vi "rsidr_core_global.vi"() -> ()   [LabVIEW 2020, in "Rohde&Schwarz RTx Oscilloscopes.lvlib"] (continued)
"Flags"=0, "Help"="Sets the transmission type to be triggered on.\n\nAvailable Repeated Capabilities:\nNone\n\nRemote-control command(s):\nTRIGger:A:MILStd:TTYPe"}, {"Level"=3, "Class Only"=FALSE, "Identifier"="RSRTX_ATTR_MILSTD_TRIGGER_FRAME", "Descriptive Name"="MILSTD Trigger Frame", "Data Type"=0, "Command"="TRIG:A:MILS:FRAM", "Access"=2, "Range Table"="RsRtx_rngMILSTDTriggerFrame", "Read Callback"="", "Write Callback"="", "Supported Models"="RTM|RTA", "Instrument Options"="", "Flags"=0, "Help"="Configures trigger frame.\n\nAvailable Repeated Capabilities:\nNone\n\nRemote-control command(s):\nTRIGger:A:MILStd:FRAMe"}, {"Level"=3, "Class Only"=TRUE, "Identifier"="", "Descriptive Name"="Error", "Data Type"=0, "Command"="", "Access"=0, "Range Table"="", "Read Callback"="", "Write Callback"="", "Supported Models"="", "Instrument Options"="", "Flags"=0, "Help"="Triggers on any combination of protocol errors. You can enable triggering on a specific type of error."}, {"Level"=4, "Class Only"=FALSE, "Identifier"="RSRTX_ATTR_MILSTD_TRIGGER_SYNCHRONIZATION_ERROR", "Descriptive Name"="MILSTD Trigger Synchronization Error", "Data Type"=3, "Command"="TRIG:A:MILS:ERR:SYNC", "Access"=2, "Range Table"="", "Read Callback"="", "Write Callback"="", "Supported Models"="RTM|RTA", "Instrument Options"="", "Flags"=0, "Help"="Enables/disables triggering when a sync impulse doesn&apos;t fulfil the technical requirements or when the transmission is not valid.\n\nAvailable Repeated Capabilities:\nNone\n\nRemote-control command(s):\nTRIGger:A:MILStd:ERRor:SYNC"}, {"Level"=4, "Class Only"=FALSE, "Identifier"="RSRTX_ATTR_MILSTD_TRIGGER_TIMEOUT_ERROR", "Descriptive Name"="MILSTD Trigger Timeout Error", "Data Type"=3, "Command"="TRIG:A:MILS:ERR:TIM", "Access"=2, "Range Table"="", "Read Callback"="", "Write Callback"="", "Supported Models"="RTM|RTA", "Instrument Options"="", "Flags"=0, "Help"="Enables/ disables triggering when the timeout is out of the set range.\n\nAvailable Repeated Capabilities:\nNone\n\nRemote-control command(s):\nTRIGger:A:MILStd:ERRor:TIMeout"}, {"Level"=4, "Class Only"=FALSE, "Identifier"="RSRTX_ATTR_MILSTD_TRIGGER_PARITY_ERROR", "Descriptive Name"="MILSTD Trigger Parity Error", "Data Type"=3, "Command"="TRIG:A:MILS:ERR:PAR", "Access"=2, "Range Table"="", "Read Callback"="", "Write Callback"="", "Supported Models"="RTM|RTA", "Instrument Options"="", "Flags"=0, "Help"="Enables/disables triggering when the parity is even.\n\nAvailable Repeated Capabilities:\nNone\n\nRemote-control command(s):\nTRIGger:A:MILStd:ERRor:PARity"}, {"Level"=4, "Class Only"=FALSE, "Identifier"="RSRTX_ATTR_MILSTD_TRIGGER_MANCHESTER_ERROR", "Descriptive Name"="MILSTD Trigger Manchester Error", "Data Type"=3, "Command"="TRIG:A:MILS:ERR:MANC", "Access"=2, "Range Table"="", "Read Callback"="", "Write Callback"="", "Supported Models"="RTM|RTA", "Instrument Options"="", "Flags"=0, "Help"="Enables/disables triggering if there is an error in the Manchester coding of the signal.\n\nAvailable Repeated Capabilities:\nNone\n\nRemote-control command(s):\nTRIGger:A:MILStd:ERRor:MANChester"}, {"Level"=3, "Class Only"=TRUE, "Identifier"="", "Descriptive Name"="Command", "Data Type"=0, "Command"="", "Access"=0, "Range Table"="", "Read Callback"="", "Write Callback"="", "Supported Models"="", "Instrument Options"="", "Flags"=0, "Help"="Triggers on any combination of protocol errors. You can enable triggering on a specific type of error."}, {"Level"=4, "Class Only"=FALSE, "Identifier"="RSRTX_ATTR_MILSTD_TRIGGER_COMMAND_TYPE", "Descriptive Name"="MILSTD Trigger Command Type", "Data Type"=0, "Command"="TRIG:A:MILS:COMM:TYPE", "Access"=2, "Range Table"="rsrtx_rngMILSTDTriggerCommandType", "Read Callback"="", "Write Callback"="", "Supported Models"="RTM|RTA", "Instrument Options"="", "Flags"=0, "Help"="Triggers on a command type.\n\nAvailable Repeated Capabilities:\nNone\n\nRemote-control command(s):\nTRIGger:A:MILStd:COMMand:TYPE"}, {"Level"=4, "Class Only"=FALSE, "Identifier"="RSRTX_ATTR_MILSTD_TRIGGER_COMMAND_DATA_DIRECTION", "Descriptive Name"="MILSTD Trigger Command Data Direction", "Data Type"=0, "Command"="TRIG:A:MILS:TRM", "Access"=2, "Range Table"="rsrtx_rngMILSTDDirection", "Read Callback"="", "Write Callback"="", "Supported Models"="RTM|RTA", "Instrument Options"="", "Flags"=0, "Help"="Triggers on a command type.\n\nAvailable Repeated Capabilities:\nNone\n\nRemote-control command(s):\nTRIGger:A:MILStd:TRMode"}, {"Level"=4, "Class Only"=FALSE, "Identifier"="RSRTX_ATTR_MILSTD_TRIGGER_RT_ADDRESS_CONDITION", "Descriptive Name"="MILSTD Trigger RT Address Condition", "Data Type"=0, "Command"="TRIG:A:MILS:RTAD:COND", "Access"=2, "Range Table"="rsrtx_rngMILSTDCondition", "Read Callback"="", "Write Callback"="", "Supported Models"="RTM|RTA", "Instrument Options"="", "Flags"=0, "Help"="For the RT address, sets the triggering condition for the comparison of the decoded value to the defined range.\n\nAvailable Repeated Capabilities:\nNone\n\nRemote-control command(s):\nTRIGger:A:MILStd:RTADdress:CONDition"}, {"Level"=4, "Class Only"=FALSE, "Identifier"="RSRTX_ATTR_MILSTD_TRIGGER_RT_ADDRESS_MINIMUM", "Descriptive Name"="MILSTD Trigger RT Address Minimum", "Data Type"=2, "Command"="TRIG:A:MILS:RTAD:MIN", "Access"=2, "Range Table"="", "Read Callback"="", "Write Callback"="", "Supported Models"="RTM|RTA", "Instrument Options"="", "Flags"=0, "Help"="Sets the minimum RT address. \n01X-string\n\nAvailable Repeated Capabilities:\nNone\n\nRemote-control command(s):\nTRIGger:A:MILStd:RTADdress:MINimum"}, {"Level"=4, "Class Only"=FALSE, "Identifier"="RSRTX_ATTR_MILSTD_TRIGGER_RT_ADDRESS_MAXIMUM", "Descriptive Name"="MILSTD Trigger RT Address Maximum", "Data Type"=2, "Command"="TRIG:A:MILS:RTAD:MAX", "Access"=2, "Range Table"="", "Read Callback"="", "Write Callback"="", "Supported Models"="RTM|RTA", "Instrument Options"="", "Flags"=0, "Help"="Sets the maximum RT address. \n01X-string\n\nAvailable Repeated Capabilities:\nNone\n\nRemote-control command(s):\nTRIGger:A:MILStd:RTADdress:MAXimum"}, {"Level"=4, "Class Only"=FALSE, "Identifier"="RSRTX_ATTR_MILSTD_TRIGGER_SUB_ADDRESS_CONDITION", "Descriptive Name"="MILSTD Trigger Sub Address Condition", "Data Type"=0, "Command"="TRIG:A:MILS:SADD:COND", "Access"=2, "Range Table"="rsrtx_rngMILSTDCondition", "Read Callback"="", "Write Callback"="", "Supported Models"="RTM|RTA", "Instrument Options"="", "Flags"=0, "Help"="For the sub address, sets the triggering condition for the comparison of the decoded value to the defined range.\n\nAvailable Repeated Capabilities:\nNone\n\nRemote-control command(s):\nTRIGger:A:MILStd:SADDress:CONDition"}, {"Level"=4, "Class Only"=FALSE, "Identifier"="RSRTX_ATTR_MILSTD_TRIGGER_SUB_ADDRESS_MINIMUM", "Descriptive Name"="MILSTD Trigger Sub Address Minimum", "Data Type"=2, "Command"="TRIG:A:MILS:SADD:MIN", "Access"=2, "Range Table"="", "Read Callback"="", "Write Callback"="", "Supported Models"="RTM|RTA", "Instrument Options"="", "Flags"=0, "Help"="Sets the minimum Sub address. \n01X-string\n\nAvailable Repeated Capabilities:\nNone\n\nRemote-control command(s):\nTRIGger:A:MILStd:SADDress:MINimum"}, {"Level"=4, "Class Only"=FALSE, "Identifier"="RSRTX_ATTR_MILSTD_TRIGGER_SUB_ADDRESS_MAXIMUM", "Descriptive Name"="MILSTD Trigger Sub Address Maximum", "Data Type"=2, "Command"="TRIG:A:MILS:SADD:MAX", "Access"=2, "Range Table"="", "Read Callback"="", "Write Callback"="", "Supported Models"="RTM|RTA", "Instrument Options"="", "Flags"=0, "Help"="Sets the maximum Sub address. \n01X-string\n\nAvailable Repeated Capabilities:\nNone\n\nRemote-control command(s):\nTRIGger:A:MILStd:SADDress:MAXimum"}, {"Level"=4, "Class Only"=FALSE, "Identifier"="RSRTX_ATTR_MILSTD_TRIGGER_SUB_ADDRESS", "Descriptive Name"="MILSTD Trigger Sub Address", "Data Type"=0, "Command"="TRIG:A:MILS:SADD:MCAD", "Access"=2, "Range Table"="rsrtx_rngMILSTDSubAddress", "Read Callback"="", "Write Callback"="", "Supported Models"="RTM|RTA", "Instrument Options"="", "Flags"=0, "Help"="Triggers on the value of the subaddress, if RSRTX_ATTR_MILSTD_TRIGGER_COMMAND_TYPE is set to mode code.\n\nAvailable Repeated Capabilities:\nNone\n\nRemote-control command(s):\nTRIGger:A:MILStd:SADDress:MCADdress"}, {"Level"=4, "Class Only"=FALSE, "Identifier"="RSRTX_ATTR_MILSTD_TRIGGER_WORD_CONDITION", "Descriptive Name"="MILSTD Trigger Word Condition", "Data Type"=0, "Command"="TRIG:A:MILS:WCO:COND", "Access"=2, "Range Table"="rsrtx_rngMILSTDCondition", "Read Callback"="", "Write Callback"="", "Supported Models"="RTM|RTA", "Instrument Options"="", "Flags"=0, "Help"="For a command word, triggers on a word comparison condition.\n\nAvailable Repeated Capabilities:\nNone\n\nRemote-control command(s):\nTRIGger:A:MILStd:WCOunt:CONDition"}, {"Level"=4, "Class Only"=FALSE, "Identifier"="RSRTX_ATTR_MILSTD_WORD_ADDRESS_MINIMUM", "Descriptive Name"="MILSTD Trigger Word Minimum", "Data Type"=0, "Command"="TRIG:A:MILS:WCO:MIN", "Access"=2, "Range Table"="", "Read Callback"="", "Write Callback"="", "Supported Models"="RTM|RTA", "Instrument Options"="", "Flags"=0, "Help"="For a command word, triggers on a minimum word count.\n01X-string\n\nAvailable Repeated Capabilities:\nNone\n\nRemote-control command(s):\nTRIGger:A:MILStd:WCOunt:MINimum"}, {"Level"=4, "Class Only"=FALSE, "Identifier"="RSRTX_ATTR_MILSTD_WORD_ADDRESS_MAXIMUM", "Descriptive Name"="MILSTD Trigger Word Maximum", "Data Type"=0, "Command"="TRIG:A:MILS:WCO:MAX", "Access"=2, "Range Table"="", "Read Callback"="", "Write Callback"="", "Supported Models"="RTM|RTA", "Instrument Options"="", "Flags"=0, "Help"="For a command word, triggers on a maximum word count.\n01X-string\n\nAvailable Repeated Capabilities:\nNone\n\nRemote-control command(s):\nTRIGger:A:MILStd:WCOunt:MAXimum"}, {"Level"=4, "Class Only"=FALSE, "Identifier"="RSRTX_ATTR_MILSTD_TRIGGER_COMMAND_MODE_CODE", "Descriptive Name"="MILSTD Trigger Command Mode Code", "Data Type"=0, "Command"="TRIG:A:MILS:MCOD:CODE", "Access"=2, "Range Table"="rsrtx_rngMILSTDCodeType", "Read Callback"="", "Write Callback"="", "Supported Models"="RTM|RTA", "Instrument Options"="", "Flags"=0, "Help"="Sets a function for the mode code to be triggered on.\n\nAvailable Repeated Capabilities:\nNone\n\nRemote-control command(s):\nTRIGger:A:MILStd:MCODe:CODE"}, {"Level"=4, "Class Only"=FALSE, "Identifier"="RSRTX_ATTR_MILSTD_TRIGGER_COMMAND_MODE_VALUE", "Descriptive Name"="MILSTD Trigger Command Mode Code Value", "Data Type"=0, "Command"="TRIG:A:MILS:MCOD:VAL", "Access"=2, "Range Table"="", "Read Callback"="", "Write Callback"="", "Supported Models"="RTM|RTA", "Instrument Options"="", "Flags"=0, "Help"="Sets the value of the mode code to be triggered on.\n\nAvailable Repeated Capabilities:\nNone\n\nRemote-control command(s):\nTRIGger:A:MILStd:MCODe:VALue"}, {"Level"=3, "Class Only"=TRUE, "Identifier"="", "Descriptive Name"="Status", "Data Type"=0, "Command"="", "Access"=0, "Range Table"="", "Read Callback"="", "Write Callback"="", "Supported Models"="", "Instrument Options"="", "Flags"=0, "Help"="Triggers on a status word that is specified."}, {"Level"=4, "Class Only"=FALSE, "Identifier"="RSRTX_ATTR_MILSTD_TRIGGER_RECEIVED_BIT_STATUS", "Descriptive Name"="MILSTD Trigger Received Bit Status", "Data Type"=0, "Command"="TRIG:A:MILS:STAT:BCR", "Access"=2, "Range Table"="rsrtx_rngStatus", "Read Callback"="", "Write Callback"="", "Supported Models"="RTM|RTA", "Instrument Options"="", "Flags"=0, "Help"="Triggers on the state of the broadcast command received bit of the status word.\n01X-string\n\nAvailable Repeated Capabilities:\nNone\n\nRemote-control command(s):\nTRIGger:A:MILStd:STATus:BCReceived"}, {"Level"=4, "Class Only"=FALSE, "Identifier"="RSRTX_ATTR_MILSTD_TRIGGER_BUSY_BIT_STATUS", "Descriptive Name"="MILSTD Trigger Busy Bit Status", "Data Type"=0, "Command"="TRIG:A:MILS:STAT:BUSY", "Access"=2, "Range Table"="rsrtx_rngStatus", "Read Callback"="", "Write Callback"="", "Supported Models"="RTM|RTA", "Instrument Options"="", "Flags"=0, "Help"="Triggers on the state of the busy bit of the status word.\n01X-string\n\nAvailable Repeated Capabilities:\nNone\n\nRemote-control command(s):\nTRIGger:A:MILStd:STATus:BUSY"}, {"Level"=4, "Class Only"=FALSE, "Identifier"="RSRTX_ATTR_MILSTD_TRIGGER_BUS_CONTROL_BIT_STATUS", "Descriptive Name"="MILSTD Trigger Bus Control Bit Status", "Data Type"=0, "Command"="TRIG:A:MILS:STAT:DBC", "Access"=2, "Range Table"="rsrtx_rngStatus", "Read Callback"="", "Write Callback"="", "Supported Models"="RTM|RTA", "Instrument Options"="", "Flags"=0, "Help"="Triggers on the state of the dynamic bus control accept bit of the status word.\n01X-string\n\nAvailable Repeated Capabilities:\nNone\n\nRemote-control command(s):\nTRIGger:A:MILStd:STATus:DBCaccept"}, {"Level"=4, "Class Only"=FALSE, "Identifier"="RSRTX_ATTR_MILSTD_TRIGGER_INSTRUMENTATION_BIT_STATUS", "Descriptive Name"="MILSTD Trigger Instrumentation Bit Status", "Data Type"=0, "Command"="TRIG:A:MILS:STAT:INST", "Access"=2, "Range Table"="rsrtx_rngStatus", "Read Callback"="", "Write Callback"="", "Supported Models"="RTM|RTA", "Instrument Options"="", "Flags"=0, "Help"="Triggers on the state of the instrumentation bit of the status word.\n01X-string\n\nAvailable Repeated Capabilities:\nNone\n\nRemote-control command(s):\nTRIGger:A:MILStd:STATus:INSTrument"}, {"Level"=4, "Class Only"=FALSE, "Identifier"="RSRTX_ATTR_MILSTD_TRIGGER_MESSAGE_ERROR_BIT_STATUS", "Descriptive Name"="MILSTD Trigger Message Error Bit Status", "Data Type"=0, "Command"="TRIG:A:MILS:STAT:MERR", "Access"=2, "Range Table"="rsrtx_rngStatus", "Read Callback"="", "Write Callback"="", "Supported Models"="RTM|RTA", "Instrument Options"="", "Flags"=0, "Help"="Triggers on the state of the message error bit of the status word.\n01X-string\n\nAvailable Repeated Capabilities:\nNone\n\nRemote-control command(s):\nTRIGger:A:MILStd:STATus:MERRor"}, {"Level"=4, "Class Only"=FALSE, "Identifier"="RSRTX_ATTR_MILSTD_TRIGGER_SERVICE_REQUEST_BIT_STATUS", "Descriptive Name"="MILSTD Trigger Service Request Bit Status", "Data Type"=0, "Command"="TRIG:A:MILS:STAT:SREQ", "Access"=2, "Range Table"="rsrtx_rngStatus", "Read Callback"="", "Write Callback"="", "Supported Models"="RTM|RTA", "Instrument Options"="", "Flags"=0, "Help"="Triggers on the state of the service request bit of the status word.\n01X-string\n\nAvailable Repeated Capabilities:\nNone\n\nRemote-control command(s):\nTRIGger:A:MILStd:STATus:SREQuest"}, {"Level"=4, "Class Only"=FALSE, "Identifier"="RSRTX_ATTR_MILSTD_TRIGGER_SUBSYSTEM_BIT_STATUS", "Descriptive Name"="MILSTD Trigger Subsystem Bit Status", "Data Type"=0, "Command"="TRIG:A:MILS:STAT:SUBS", "Access"=2, "Range Table"="rsrtx_rngStatus", "Read Callback"="", "Write Callback"="", "Supported Models"="RTM|RTA", "Instrument Options"="", "Flags"=0, "Help"="Triggers on the state of the subsystem flag bit of the status word.\n01X-string\n\nAvailable Repeated Capabilities:\nNone\n\nRemote-control command(s):\nTRIGger:A:MILStd:STATus:SUBSystem"}, {"Level"=4, "Class Only"=FALSE, "Identifier"="RSRTX_ATTR_MILSTD_TRIGGER_TERMINAL_BIT_STATUS", "Descriptive Name"="MILSTD Trigger Terminal Bit Status", "Data Type"=0, "Command"="TRIG:A:MILS:STAT:TERM", "Access"=2, "Range Table"="rsrtx_rngStatus", "Read Callback"="", "Write Callback"="", "Supported Models"="RTM|RTA", "Instrument Options"="", "Flags"=0, "Help"="Triggers on the state of the terminal flag bit of the status word.\n01X-string\n\nAvailable Repeated Capabilities:\nNone\n\nRemote-control command(s):\nTRIGger:A:MILStd:STATus:TERMinal"}, {"Level"=3, "Class Only"=TRUE, "Identifier"="", "Descriptive Name"="Data", "Data Type"=0, "Command"="", "Access"=0, "Range Table"="", "Read Callback"="", "Write Callback"="", "Supported Models"="", "Instrument Options"="", "Flags"=0, "Help"="Triggers on a data, that is specified."}, {"Level"=4, "Class Only"=FALSE, "Identifier"="RSRTX_ATTR_MILSTD_TRIGGER_DATA_CONDITION", "Descriptive Name"="MILSTD Trigger Data Condition", "Data Type"=0, "Command"="TRIG:A:MILS:DATA:COND", "Access"=2, "Range Table"="rsrtx_rngMILSTDCondition", "Read Callback"="", "Write Callback"="", "Supported Models"="RTM|RTA", "Instrument Options"="", "Flags"=0, "Help"="For a data word, sets the triggering condition for the comparison of the decoded value to the defined range.\n\nAvailable Repeated Capabilities:\nNone\n\nRemote-control command(s):\nTRIGger:A:MILStd:DATA:CONDition"}, {"Level"=4, "Class Only"=FALSE, "Identifier"="RSRTX_ATTR_MILSTD_TRIGGER_DATA_MINIMUM", "Descriptive Name"="MILSTD Trigger Data Minimum", "Data Type"=2, "Command"="TRIG:A:MILS:DATA:MIN", "Access"=2, "Range Table"="", "Read Callback"="", "Write Callback"="", "Supported Models"="RTM|RTA", "Instrument Options"="", "Flags"=0, "Help"="For a data word, sets the minimum data value.\n01X-string\n\nAvailable Repeated Capabilities:\nNone\n\nRemote-control command(s):\nTRIGger:A:MILStd:DATA:MINimum"}, {"Level"=4, "Class Only"=FALSE, "Identifier"="RSRTX_ATTR_MILSTD_TRIGGER_DATA_MAXIMUM", "Descriptive Name"="MILSTD Trigger Data Maximum", "Data Type"=2, "Command"="TRIG:A:MILS:DATA:MAX", "Access"=2, "Range Table"="", "Read Callback"="", "Write Callback"="", "Supported Models"="RTM|RTA", "Instrument Options"="", "Flags"=0, "Help"="For a data word, sets the maximum data value. \n01X-string\n\nAvailable Repeated Capabilities:\nNone\n\nRemote-control command(s):\nTRIGger:A:MILStd:DATA:MAXimum"}, {"Level"=4, "Class Only"=FALSE, "Identifier"="RSRTX_ATTR_MILSTD_TRIGGER_DATA_OFFSET_CONDITION", "Descriptive Name"="MILSTD Trigger Data Offset Condition", "Data Type"=0, "Command"="TRIG:A:MILS:DATA:OFFS:COND", "Access"=2, "Range Table"="rsrtx_rngMILSTDCondition", "Read Callback"="", "Write Callback"="", "Supported Models"="RTM|RTA", "Instrument Options"="", "Flags"=0, "Help"="For a data offset, sets the triggering condition for the comparison of the decoded value to the defined range.\n\nAvailable Repeated Capabilities:\nNone\n\nRemote-control command(s):\nTRIGger:A:MILStd:DATA:OFFSet:CONDition"}, {"Level"=4, "Class Only"=FALSE, "Identifier"="RSRTX_ATTR_MILSTD_TRIGGER_DATA_OFFSET", "Descriptive Name"="MILSTD Trigger Data Offset", "Data Type"=0, "Command"="TRIG:A:MILS:DATA:OFFS", "Access"=2, "Range Table"="", "Read Callback"="", "Write Callback"="", "Supported Models"="RTM|RTA", "Instrument Options"="", "Flags"=0, "Help"="For a data word sets the word offset to be triggered on.\n\nAvailable Repeated Capabilities:\nNone\n\nRemote-control command(s):\nTRIGger:A:MILStd:DATA:OFFSet"}, {"Level"=4, "Class Only"=FALSE, "Identifier"="RSRTX_ATTR_MILSTD_TRIGGER_DATA_OFFSET_WORDS", "Descriptive Name"="MILSTD Trigger Data Offset Words", "Data Type"=0, "Command"="TRIG:A:MILS:DATA:WORD", "Access"=2, "Range Table"="", "Read Callback"="", "Write Callback"="", "Supported Models"="RTM|RTA", "Instrument Options"="", "Flags"=0, "Help"="For a data word sets the number of words to be triggered on.\n\nAvailable Repeated Capabilities:\nNone\n\nRemote-control command(s):\nTRIGger:A:MILStd:DATA:WORDs"}, {"Level"=2, "Class Only"=TRUE, "Identifier"="", "Descriptive Name"="ARINC 429", "Data Type"=0, "Command"="", "Access"=0, "Range Table"="", "Read Callback"="", "Write Callback"="", "Supported Models"="", "Instrument Options"="", "Flags"=0, "Help"="Configures ARINC 429 trigger settings."}, {"Level"=3, "Class Only"=FALSE, "Identifier"="RSRTX_ATTR_PROTOCOL_ARINC429_TRIGGER_TYPE", "Descriptive Name"="Protocol ARINC429 Trigger Type", "Data Type"=0, "Command"="TRIG:A:ARIN:TYPE", "Access"=2, "Range Table"="rsrtx_rngARINC429Type", "Read Callback"="", "Write Callback"="", "Supported Models"="RTM|RTA", "Instrument Options"="", "Flags"=0, "Help"="Selects the type of trigger.\n\nAvailable Repeated Capabilities:\nNone\n\nRemote-control command(s):\nTRIGger:A:ARINc:TYPE"}, {"Level"=3, "Class Only"=FALSE, "Identifier"="RSRTX_ATTR_PROTOCOL_ARINC429_TRIGGER_WORD_TYPE", "Descriptive Name"="Protocol ARINC429 Trigger Word Type", "Data Type"=0, "Command"="TRIG:A:ARIN:WORD:TYPE", "Access"=2, "Range Table"="rsrtx_rngARINC429WordType", "Read Callback"="", "Write Callback"="", "Supported Models"="RTM|RTA", "Instrument Options"="", "Flags"=0, "Help"="Sets the word type to be triggered on.\n\nAvailable Repeated Capabilities:\nNone\n\nRemote-control command(s):\nTRIGger:A:ARINc:WORD:TYPE"}, {"Level"=3, "Class Only"=TRUE, "Identifier"="", "Descriptive Name"="Error Condition", "Data Type"=0, "Command"="", "Access"=0, "Range Table"="", "Read Callback"="", "Write Callback"="", "Supported Models"="", "Instrument Options"="", "Flags"=0, "Help"="Specifies the error conditions to be triggered on."}, {"Level"=4, "Class Only"=FALSE, "Identifier"="RSRTX_ATTR_PROTOCOL_ARINC429_TRIGGER_ERROR_CODING_ERROR", "Descriptive Name"="Protocol ARINC429 Trigger Error Coding Error", "Data Type"=3, "Command"="TRIG:A:ARIN:ERR:COD", "Access"=2, "Range Table"="", "Read Callback"="", "Write Callback"="", "Supported Models"="RTM|RTA", "Instrument Options"="", "Flags"=0, "Help"="Enables triggering when a coding error occurs.\n\nAvailable Repeated Capabilities:\nNone\n\nRemote-control command(s):\nTRIGger:A:ARINc:ERRor:CODing"}, {"Level"=4, "Class Only"=FALSE, "Identifier"="RSRTX_ATTR_PROTOCOL_ARINC429_TRIGGER_ERROR_PARITY_ERROR", "Descriptive Name"="Protocol ARINC429 Trigger Error Parity Error", "Data Type"=3, "Command"="TRIG:A:ARIN:ERR:PAR", "Access"=2, "Range Table"="", "Read Callback"="", "Write Callback"="", "Supported Models"="RTM|RTA", "Instrument Options"="", "Flags"=0, "Help"="Enables triggering when a parity error occurs.\n\nAvailable Repeated Capabilities:\nNone\n\nRemote-control command(s):\nTRIGger:A:ARINc:ERRor:PARity"}, {"Level"=4, "Class Only"=FALSE, "Identifier"="RSRTX_ATTR_PROTOCOL_ARINC429_TRIGGER_ERROR_GAP_ERROR", "Descriptive Name"="Protocol ARINC429 Trigger Error Gap Error", "Data Type"=3, "Command"="TRIG:A:ARIN:ERR:GAP", "Access"=2, "Range Table"="", "Read Callback"="", "Write Callback"="", "Supported Models"="RTM|RTA", "Instrument Options"="", "Flags"=0, "Help"="Enables triggering when a gap error occurs.\n\nAvailable Repeated Capabilities:\nNone\n\nRemote-control command(s):\nTRIGger:A:ARINc:ERRor:GAP"}, {"Level"=3, "Class Only"=TRUE, "Identifier"="", "Descriptive Name"="Label Data", "Data Type"=0, "Command"="", "Access"=0, "Range Table"="", "Read Callback"="", "Write Callback"="", "Supported Models"="", "Instrument Options"="", "Flags"=0, "Help"="Configures ARINC 429 trigger label+data settings."}, {"Level"=4, "Class Only"=FALSE, "Identifier"="RSRTX_ATTR_PROTOCOL_ARINC429_TRIGGER_LABEL_DATA_SDI", "Descriptive Name"="Protocol ARINC429 Trigger Label Data SDI", "Data Type"=0, "Command"="TRIG:A:ARIN:SDI", "Access"=2, "Range Table"="rsrtx_rngARINCSsmSdi", "Read Callback"="", "Write Callback"="", "Supported Models"="RTM|RTA", "Instrument Options"="", "Flags"=0, "Help"="Sets the source/destination identifier (SDI) bits.\n\nAvailable Repeated Capabilities:\nNone\n\nRemote-control command(s):\nTRIGger:A:ARINc:SDI"}, {"Level"=4, "Class Only"=FALSE, "Identifier"="RSRTX_ATTR_PROTOCOL_ARINC429_TRIGGER_LABEL_DATA_SSM", "Descriptive Name"="Protocol ARINC429 Trigger Label Data SSM", "Data Type"=0, "Command"="TRIG:A:ARIN:SSM", "Access"=2, "Range Table"="rsrtx_rngARINCSsmSdi", "Read Callback"="", "Write Callback"="", "Supported Models"="RTM|RTA", "Instrument Options"="", "Flags"=0, "Help"="Sets the sign/status matrix (SSM) bits.\n\nAvailable Repeated Capabilities:\nNone\n\nRemote-control command(s):\nTRIGger:A:ARINc:SSM"}, {"Level"=4, "Class Only"=FALSE, "Identifier"="RSRTX_ATTR_PROTOCOL_ARINC429_TRIGGER_LABEL_DATA_FORMAT", "Descriptive Name"="Protocol ARINC429 Trigger Label Data Format", "Data Type"=0, "Command"="TRIG:A:ARIN:FORM", "Access"=2, "Range Table"="rsrtx_rngProtocolARINC429DataFormat", "Read Callback"="", "Write Callback"="", "Supported Models"="RTM|RTA", "Instrument Options"="", "Flags"=0, "Help"="Sets the the transmission format to be triggered on.\n\nAvailable Repeated Capabilities:\nNone\n\nRemote-control command(s):\nTRIGger:A:ARINc:FORMat"}, {"Level"=4, "Class Only"=FALSE, "Identifier"="RSRTX_ATTR_PROTOCOL_ARINC429_TRIGGER_LABEL_PATTERN_CONDITION", "Descriptive Name"="Protocol ARINC429 Trigger Label Pattern Condition", "Data Type"=0, "Command"="TRIG:A:ARIN:LAB:COND", "Access"=2, "Range Table"="rsrtx_rngProtocolARINC429Operator", "Read Callback"="", "Write Callback"="", "Supported Models"="RTM|RTA", "Instrument Options"="", "Flags"=0, "Help"="Sets the condition for the label. You can define an exact label or a label range.\n\nAvailable Repeated Capabilities:\nNone\n\nRemote-control command(s):\nTRIGger:A:ARINc:LABel:CONDition"}, {"Level"=4, "Class Only"=FALSE, "Identifier"="RSRTX_ATTR_PROTOCOL_ARINC429_TRIGGER_LABEL_PATTERN_MIN", "Descriptive Name"="Protocol ARINC429 Trigger Label Pattern Min", "Data Type"=2, "Command"="TRIG:A:ARIN:LAB:MIN", "Access"=2, "Range Table"="", "Read Callback"="", "Write Callback"="", "Supported Models"="RTM|RTA", "Instrument Options"="", "Flags"=0, "Help"="Defines the minimum bit pattern for the label.\n\nAvailable Repeated Capabilities:\nNone\n\nRemote-control command(s):\nTRIGger:A:ARINc:LABel:MINimum"}, {"Level"=4, "Class Only"=FALSE, "Identifier"="RSRTX_ATTR_PROTOCOL_ARINC429_TRIGGER_LABEL_PATTERN_MAX", "Descriptive Name"="Protocol ARINC429 Trigger Label Pattern Max", "Data Type"=2, "Command"="TRIG:A:ARIN:LAB:MAX", "Access"=2, "Range Table"="", "Read Callback"="", "Write Callback"="", "Supported Models"="RTM|RTA", "Instrument Options"="", "Flags"=0, "Help"="Sets the end value of a label pattern if Label Pattern Condition is set to InRange or OutOfRange.\n\nAvailable Repeated Capabilities:\nNone\n\nRemote-control command(s):\nTRIGger:A:ARINc:LABel:MAXimum"}, {"Level"=4, "Class Only"=FALSE, "Identifier"="RSRTX_ATTR_PROTOCOL_ARINC429_TRIGGER_DATA_PATTERN_CONDITION", "Descriptive Name"="Protocol ARINC429 Trigger Data Pattern Condition", "Data Type"=0, "Command"="TRIG:A:ARIN:DATA:COND", "Access"=2, "Range Table"="rsrtx_rngProtocolARINC429Operator", "Read Callback"="", "Write Callback"="", "Supported Models"="RTM|RTA", "Instrument Options"="", "Flags"=0, "Help"="Define the operators for comparison of the decoded data condition with the specified data.\n\nAvailable Repeated Capabilities:\nNone\n\nRemote-control command(s):\nTRIGger:A:ARINc:DATA:CONDition"}, {"Level"=4, "Class Only"=FALSE, "Identifier"="RSRTX_ATTR_PROTOCOL_ARINC429_TRIGGER_DATA_PATTERN_MIN", "Descriptive Name"="Protocol ARINC429 Trigger Data Pattern Min", "Data Type"=2, "Command"="TRIG:A:ARIN:DATA:MIN", "Access"=2, "Range Table"="", "Read Callback"="", "Write Callback"="", "Supported Models"="RTM|RTA", "Instrument Options"="", "Flags"=0, "Help"="Defines the minimum bit pattern for the data.\n\nAvailable Repeated Capabilities:\nNone\n\nRemote-control command(s):\nTRIGger:A:ARINc:DATA:MINimum"}, {"Level"=4, "Class Only"=FALSE, "Identifier"="RSRTX_ATTR_PROTOCOL_ARINC429_TRIGGER_DATA_PATTERN_MAX", "Descriptive Name"="Protocol ARINC429 Trigger Data Pattern Max", "Data Type"=2, "Command"="TRIG:A:ARIN:DATA:MAX", "Access"=2, "Range Table"="", "Read Callback"="", "Write Callback"="", "Supported Models"="RTM|RTA", "Instrument Options"="", "Flags"=0, "Help"="Sets the end value of a data pattern if Data Pattern Condition is set to InRange or OutOfRange.\n\nAvailable Repeated Capabilities:\nNone\n\nRemote-control command(s):\nTRIGger:A:ARINc:DATA:MAXimum"}, {"Level"=4, "Class Only"=FALSE, "Identifier"="RSRTX_ATTR_PROTOCOL_ARINC429_TRIGGER_DATA_OFFSET", "Descriptive Name"="Protocol ARINC429 Trigger Data Offset", "Data Type"=0, "Command"="TRIG:A:ARIN:DATA:OFFS", "Access"=2, "Range Table"="", "Read Callback"="", "Write Callback"="", "Supported Models"="RTM|RTA", "Instrument Options"="", "Flags"=0, "Help"="Sets a data offset.\n\nAvailable Repeated Capabilities:\nNone\n\nRemote-control command(s):\nTRIGger:A:ARINc:DATA:OFFSet"}, {"Level"=4, "Class Only"=FALSE, "Identifier"="RSRTX_ATTR_PROTOCOL_ARINC429_TRIGGER_DATA_SIZE", "Descriptive Name"="Protocol ARINC429 Trigger Data Size", "Data Type"=0, "Command"="TRIG:A:ARIN:DATA:SIZE", "Access"=2, "Range Table"="", "Read Callback"="", "Write Callback"="", "Supported Models"="RTM|RTA", "Instrument Options"="", "Flags"=0, "Help"="Sets the data size.\n\nAvailable Repeated Capabilities:\nNone\n\nRemote-control command(s):\nTRIGger:A:ARINc:DATA:SIZE"}, {"Level"=3, "Class Only"=TRUE, "Identifier"="", "Descriptive Name"="Timing", "Data Type"=0, "Command"="", "Access"=0, "Range Table"="", "Read Callback"="", "Write Callback"="", "Supported Models"="", "Instrument Options"="", "Flags"=0, "Help"="Specifies the timeouts to be triggered on."}, {"Level"=4, "Class Only"=FALSE, "Identifier"="RSRTX_ATTR_PROTOCOL_ARINC429_TRIGGER_TIMING_CONDITION", "Descriptive Name"="Protocol ARINC429 Trigger Timing Condition", "Data Type"=0, "Command"="TRIG:A:ARIN:TTIM:COND", "Access"=2, "Range Table"="rsrtx_rngARINC429TimingCondition", "Read Callback"="", "Write Callback"="", "Supported Models"="RTM|RTA", "Instrument Options"="", "Flags"=0, "Help"="Define the operators for comparison of the decoded transmission time condition with the specified data.\n\nAvailable Repeated Capabilities:\nNone\n\nRemote-control command(s):\nTRIGger:A:ARINc:TTIMe:CONDition"}, {"Level"=4, "Class Only"=FALSE, "Identifier"="RSRTX_ATTR_PROTOCOL_ARINC429_TRIGGER_TIMING_MIN", "Descriptive Name"="Protocol ARINC429 Trigger Timing Min", "Data Type"=1, "Command"="TRIG:A:ARIN:TTIM:MIN", "Access"=2, "Range Table"="", "Read Callback"="", "Write Callback"="", "Supported Models"="RTM|RTA", "Instrument Options"="", "Flags"=0, "Help"="Sets the minimum value of the transmission time.\n\nAvailable Repeated Capabilities:\nNone\n\nRemote-control command(s):\nTRIGger:A:ARINc:TTIMe:MINimum"}, {"Level"=4, "Class Only"=FALSE, "Identifier"="RSRTX_ATTR_PROTOCOL_ARINC429_TRIGGER_TIMING_MAX", "Descriptive Name"="Protocol ARINC429 Trigger Timing Max", "Data Type"=1, "Command"="TRIG:A:ARIN:TTIM:MAX", "Access"=2, "Range Table"="", "Read Callback"="", "Write Callback"="", "Supported Models"="RTM|RTA", "Instrument Options"="", "Flags"=0, "Help"="Sets the maximu value of the transmission time.\n\nAvailable Repeated Capabilities:\nNone\n\nRemote-control command(s):\nTRIGger:A:ARINc:TTIMe:MAXimum"}, {"Level"=1, "Class Only"=TRUE, "Identifier"="", "Descriptive Name"="Waveform Acquisition", "Data Type"=0, "Command"="", "Access"=0, "Range Table"="", "Read Callback"="", "Write Callback"="", "Supported Models"="", "Instrument Options"="", "Flags"=0, "Help"="Attributes that configure the waveform measurement."}, {"Level"=2, "Class Only"=FALSE, "Identifier"="RSRTX_ATTR_RUN_SINGLE", "Descriptive Name"="Run Single", "Data Type"=4, "Command"="SING", "Access"=1, "Range Table"="", "Read Callback"="", "Write Callback"="", "Supported Models"="", "Instrument Options"="", "Flags"=0, "Help"="Starts a defined number of acquisition cycles.\n\nAvailable Repeated Capabilities:\nNone\n\nRemote-control command(s):\nSINGle"}, {"Level"=2, "Class Only"=FALSE, "Identifier"="RSRTX_ATTR_RUN_SINGLE_WAIT_FOR_OPC", "Descriptive Name"="Run Single Wait For OPC", "Data Type"=4, "Command"="SING", "Access"=1, "Range Table"="", "Read Callback"="", "Write Callback"="", "Supported Models"="", "Instrument Options"="", "Flags"=1, "Help"="Starts a defined number of acquisition cycles.\n\nAvailable Repeated Capabilities:\nNone\n\nRemote-control command(s):\nSINGle"}, {"Level"=2, "Class Only"=FALSE, "Identifier"="RSRTX_ATTR_RUN_CONTINUOUS", "Descriptive Name"="Run Continuous", "Data Type"=4, "Command"="RUN", "Access"=1, "Range Table"="", "Read Callback"="", "Write Callback"="", "Supported Models"="", "Instrument Options"="", "Flags"=0, "Help"="Starts the continuous acquisition.\n\nAvailable Repeated Capabilities:\nNone\n\nRemote-control command(s):\nRUN"}, {"Level"=2, "Class Only"=FALSE, "Identifier"="RSRTX_ATTR_STOP", "Descriptive Name"="Stop", "Data Type"=4, "Command"="STOP", "Access"=1, "Range Table"="", "Read Callback"="", "Write Callback"="", "Supported Models"="", "Instrument Options"="", "Flags"=0, "Help"="Stops the running acquistion.\n\nAvailable Repeated Capabilities:\nNone\n\nRemote-control command(s):\nSTOP"}, {"Level"=2, "Class Only"=FALSE, "Identifier"="RSRTX_ATTR_SEND_SW_TRIGGER", "Descriptive Name"="Send SW Trigger", "Data Type"=4, "Command"="*TRG", "Access"=1, "Range Table"="", "Read Callback"="", "Write Callback"="", "Supported Models"="", "Instrument Options"="", "Flags"=1, "Help"="Triggers all actions waiting for a trigger event. In particular, *TRG generates a manual trigger signal (Manual Trigger).\n\nAvailable Repeated Capabilities:\nNone\n\nRemote-control command(s):\n*TRG"}, {"Level"=2, "Class Only"=FALSE, "Identifier"="RSRTX_ATTR_ACQUISITION_STATE", "Descriptive Name"="Acquisition State", "Data Type"=0, "Command"="ACQ:STAT", "Access"=2, "Range Table"="RsRtx_rngAcquisitionState", "Read Callback"="", "Write Callback"="", "Supported Models"="", "Instrument Options"="", "Flags"=0, "Help"="Sets or queries the acquisition state of the instrument.\n\nAvailable Repeated Capabilities:\nNone\n\nRemote-control command(s):\nACQuire:STATe"}, {"Level"=2, "Class Only"=TRUE, "Identifier"="", "Descriptive Name"="Waveform Export", "Data Type"=0, "Command"="", "Access"=0, "Range Table"="", "Read Callback"="", "Write Callback"="", "Supported Models"="", "Instrument Options"="", "Flags"=0, "Help"="Contains attributes for waveform exporting."}, {"Level"=3, "Class Only"=FALSE, "Identifier"="RSRTX_ATTR_WAVEFROM_EXPORT_NAME", "Descriptive Name"="Wavefrom Export Name", "Data Type"=2, "Command"="EXP:WAV:NAME", "Access"=2, "Range Table"="", "Read Callback"="", "Write Callback"="", "Supported Models"="", "Instrument Options"="", "Flags"=0, "Help"="Defines the path and filename for a waveform data file that will be saved. The file format is CSV. If the file already exists, it will be overwritten.\n\nAvailable Repeated Capabilities:\nNone\n\nRemote-control command(s):\nEXPort:WAVeform:NAME"}, {"Level"=3, "Class Only"=FALSE, "Identifier"="RSRTX_ATTR_WAVEFORM_EXPORT_SOURCE", "Descriptive Name"="Waveform Export Source", "Data Type"=0, "Command"="EXP:WAV:SOUR", "Access"=2, "Range Table"="rsrtx_rngWaveformExportParameter", "Read Callback"="", "Write Callback"="", "Supported Models"="", "Instrument Options"="", "Flags"=0, "Help"="Defines the waveform to be exported.\n\nAvailable Repeated Capabilities:\nNone\n\nRemote-control command(s):\nEXPort:WAVeform:SOURce"}, {"Level"=3, "Class Only"=FALSE, "Identifier"="RSRTX_ATTR_WAVEFORM_EXPORT_DESTINATION", "Descriptive Name"="Waveform Export Destination", "Data Type"=2, "Command"="EXP:WFMS:DEST", "Access"=2, "Range Table"="", "Read Callback"="", "Write Callback"="", "Supported Models"="", "Instrument Options"="", "Flags"=0, "Help"="Defines the directory where waveforms are saved. The specified directory must exist before the command is sent.\n\nAvailable Repeated Capabilities:\nNone\n\nRemote-control command(s):\nEXPort:WFMSave:DESTination"}, {"Level"=3, "Class Only"=FALSE, "Identifier"="RSRTX_ATTR_WAVEFORM_EXPORT_SAVE", "Descriptive Name"="Waveform Export Save", "Data Type"=4, "Command"="EXP:WAV:SAVE", "Access"=1, "Range Table"="", "Read Callback"="", "Write Callback"="", "Supported Models"="", "Instrument Options"="", "Flags"=0, "Help"="Executes saving a waveform, for which the path and filename have been defined by RSRTX_ATTR_WAVEFROM_EXPORT_NAME.\n\nAvailable Repeated Capabilities:\nNone\n\nRemote-control command(s):\nEXPort:WAVeform:SAVE"}, {"Level"=2, "Class Only"=TRUE, "Identifier"="", "Descriptive Name"="Waveform", "Data Type"=0, "Command"="", "Access"=0, "Range Table"="", "Read Callback"="", "Write Callback"="", "Supported Models"="", "Instrument Options"="", "Flags"=0, "Help"="Acquires waveform data."}, {"Level"=3, "Class Only"=FALSE, "Identifier"="RSRTX_ATTR_WAVEFORM_SAMPLES", "Descriptive Name"="Waveform Samples", "Data Type"=0, "Command"="CHAN{Channel}:DATA:POIN?", "Access"=0, "Range Table"="", "Read Callback"="", "Write Callback"="", "Supported Models"="", "Instrument Options"="", "Flags"=0, "Help"="Returns the number of samples for the selected range.\n\nAvailable Repeated Capabilities:\nChannel: CH0, CH1, CH2, CH3, CH4, CHExt\r\n\nRemote-control command(s):\nCHANnel<m>:DATA:POINts"}, {"Level"=2, "Class Only"=TRUE, "Identifier"="", "Descriptive Name"="Waveform Conversion", "Data Type"=0, "Command"="", "Access"=0, "Range Table"="", "Read Callback"="", "Write Callback"="", "Supported Models"="", "Instrument Options"="", "Flags"=0, "Help"="Attributes for conversion of waveform data."}, {"Level"=3, "Class Only"=FALSE, "Identifier"="RSRTX_ATTR_WAVEFORM_CONVERSION_X_START", "Descriptive Name"="Waveform Conversion X Start", "Data Type"=1, "Command"="CHAN{Channel}:DATA:XOR?", "Access"=0, "Range Table"="", "Read Callback"="", "Write Callback"="", "Supported Models"="", "Instrument Options"="", "Flags"=0, "Help"="Return the time of the first sample of the indicated waveform.\n\nAvailable Repeated Capabilities:\nChannel: CH0, CH1, CH2, CH3, CH4, CHExt\r\n\nRemote-control command(s):\nCHANnel<m>:DATA:XORigin?"}, {"Level"=3, "Class Only"=FALSE, "Identifier"="RSRTX_ATTR_WAVEFORM_CONVERSION_X_INCREMENT", "Descriptive Name"="Waveform Conversion X Increment", "Data Type"=1, "Command"="CHAN{Channel}:DATA:XINC?", "Access"=0, "Range Table"="", "Read Callback"="", "Write Callback"="", "Supported Models"="", "Instrument Options"="", "Flags"=0, "Help"="Return the time difference between two adjacent samples of the indicated waveform.\n\nAvailable Repeated Capabilities:\nChannel: CH0, CH1, CH2, CH3, CH4, CHExt\r\n\nRemote-control command(s):\nCHANnel<m>:DATA:XINCrement?"}, {"Level"=3, "Class Only"=FALSE, "Identifier"="RSRTX_ATTR_WAVEFORM_CONVERSION_Y_START", "Descriptive Name"="Waveform Conversion Y Start", "Data Type"=1, "Command"="CHAN{Channel}:DATA:YOR?", "Access"=0, "Range Table"="", "Read Callback"="", "Write Callback"="", "Supported Models"="", "Instrument Options"="", "Flags"=0, "Help"="Return the voltage value for binary value 0 of the indicated waveform.\n\nAvailable Repeated Capabilities:\nChannel: CH0, CH1, CH2, CH3, CH4, CHExt\r\n\nRemote-control command(s):\nCHANnel<m>:DATA:YORigin?"}, {"Level"=3, "Class Only"=FALSE, "Identifier"="RSRTX_ATTR_WAVEFORM_CONVERSION_Y_INCREMENT", "Descriptive Name"="Waveform Conversion Y Increment", "Data Type"=1, "Command"="CHAN{Channel}:DATA:YINC?", "Access"=0, "Range Table"="", "Read Callback"="", "Write Callback"="", "Supported Models"="", "Instrument Options"="", "Flags"=0, "Help"="Return the voltage value per bit of the indicated waveform.\n\nAvailable Repeated Capabilities:\nChannel: CH0, CH1, CH2, CH3, CH4, CHExt\r\n\nRemote-control command(s):\nCHANnel<m>:DATA:YINCrement?"}, {"Level"=3, "Class Only"=FALSE, "Identifier"="RSRTX_ATTR_WAVEFORM_CONVERSION_Y_RESOLUTION", "Descriptive Name"="Waveform Conversion Y Resolution", "Data Type"=0, "Command"="CHAN{Channel}:DATA:YRES?", "Access"=0, "Range Table"="", "Read Callback"="", "Write Callback"="", "Supported Models"="", "Instrument Options"="", "Flags"=0, "Help"="Return the vertical bit resolution of the indicated waveform.\n\nAvailable Repeated Capabilities:\nChannel: CH0, CH1, CH2, CH3, CH4, CHExt\r\n\nRemote-control command(s):\nCHANnel<m>:DATA:YRESolution?"}, {"Level"=2, "Class Only"=TRUE, "Identifier"="", "Descriptive Name"="Envelope Waveform", "Data Type"=0, "Command"="", "Access"=0, "Range Table"="", "Read Callback"="", "Write Callback"="", "Supported Models"="", "Instrument Options"="", "Flags"=0, "Help"="Acquires waveform data."}, {"Level"=2, "Class Only"=TRUE, "Identifier"="", "Descriptive Name"="Envelope Waveform Conversion", "Data Type"=0, "Command"="", "Access"=0, "Range Table"="", "Read Callback"="", "Write Callback"="", "Supported Models"="", "Instrument Options"="", "Flags"=0, "Help"="Attributes for conversion of envelope data."}, {"Level"=3, "Class Only"=FALSE, "Identifier"="RSRTX_ATTR_ENVELOPE_WAVEFORM_CONVERSION_X_START", "Descriptive Name"="Envelope Waveform Conversion X Start", "Data Type"=1, "Command"="CHAN{Channel}:DATA:ENV:XOR?",
